vi "AB_Load_Class.vi"(8 "error in (no error)":errorcluster, 11 "AB_Class path":path) -> (0 "error out":errorcluster, 3 "AB_Build out":refnum<class "AB_Build.lvclass">)   [LabVIEW 2020]
uses:
  <vilib>/AppBuilder/AB_Classes/Build/AB_Build.lvclass
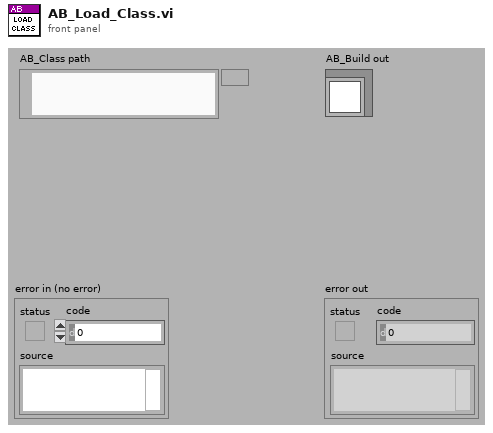
[diagram p1: front panel]
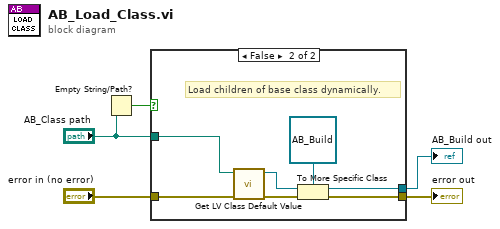
[diagram p0: block diagram]
diagram:
  n1 = Empty String/Path?(string/path="AB_Class path") -> (empty?=w2:bool)
  n2 = case shown="False" w2 {
    tunnel: [_ w13] -> w5
    tunnel: "error in (no error)" -> [w6 w12]
    tunnel: [w6 w11] -> w3
    tunnel: "AB_Class path" -> [_ w7]
    frame True {
      # "Source Distribution"
      # "If path is not valid, return default base class object."
    }
    frame False {
      # "Load children of base class dynamically."
      n3 = call <vilib>:"Get LV Class Default Value.vi"("error in (no error)"=w12, "class path"=w7) -> ("error out"=w9:errorcluster, "object"=w8:refnum<class>)  [unwired: 8 in]
      n4 = To More Specific Class(target class=refnum<class "AB_Build.lvclass"> refnum ("AB_Build out"), reference=w8, error in=w9) -> (specific class reference=w13:refnum<class "AB_Build.lvclass">, error out=w11:errorcluster)
    }
  }
  "AB_Build out" <- w5
  "error out" <- w3
